vi "外观 2.vi"(0 "Data In":T5 caption="数据输入", 2 "Display State In":T3 caption="显示状态输入", 3 "Container State":T4 caption="容器状态") -> (6 "Data Out":T5 caption="数据输出", 7 "Display State Out":T3 caption="显示状态输出", 8 "Action":T2 caption="动作")   [LabVIEW 2016, in "运维调试菜单_古田户外.xctl"]
uses:
  <vilib>/_xctls/Container State.ctl
  <vilib>/_xctls/Action.ctl
  <vilib>/_xctls/XControlSupport.lvlib
panel:
  in  "单选按钮":T1(radio)
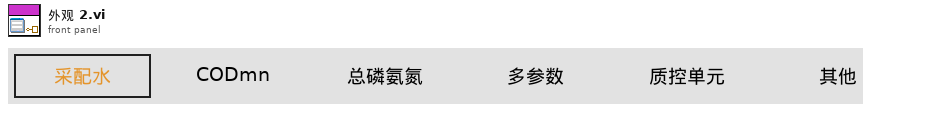
[diagram p1: front panel]
types:
  T1 = enum32{"采配水", "CODMn", "总磷氨氮", "pH", "质控单元", "其他"}
  T2 = typedef "XControlSupport.lvlib/Action.ctl" = cluster{"Data Changed?":bool, "State Changed?":bool, "Action Name":string}
  T3 = typedef "运维调试菜单_古田户外.xctl/状态 2.ctl" = cluster{"Numeric":dbl}
  T4 = typedef "XControlSupport.lvlib/Container State.ctl" = cluster{"Indicator?":bool, "Run Mode?":bool, " Refnum":refnum<vi>}
  T5 = typedef "运维调试菜单_古田户外.xctl/数据 2.ctl" = enum16{"采配水", "CODmn", "总磷氨氮", "多参数", "质控单元", "其他"}
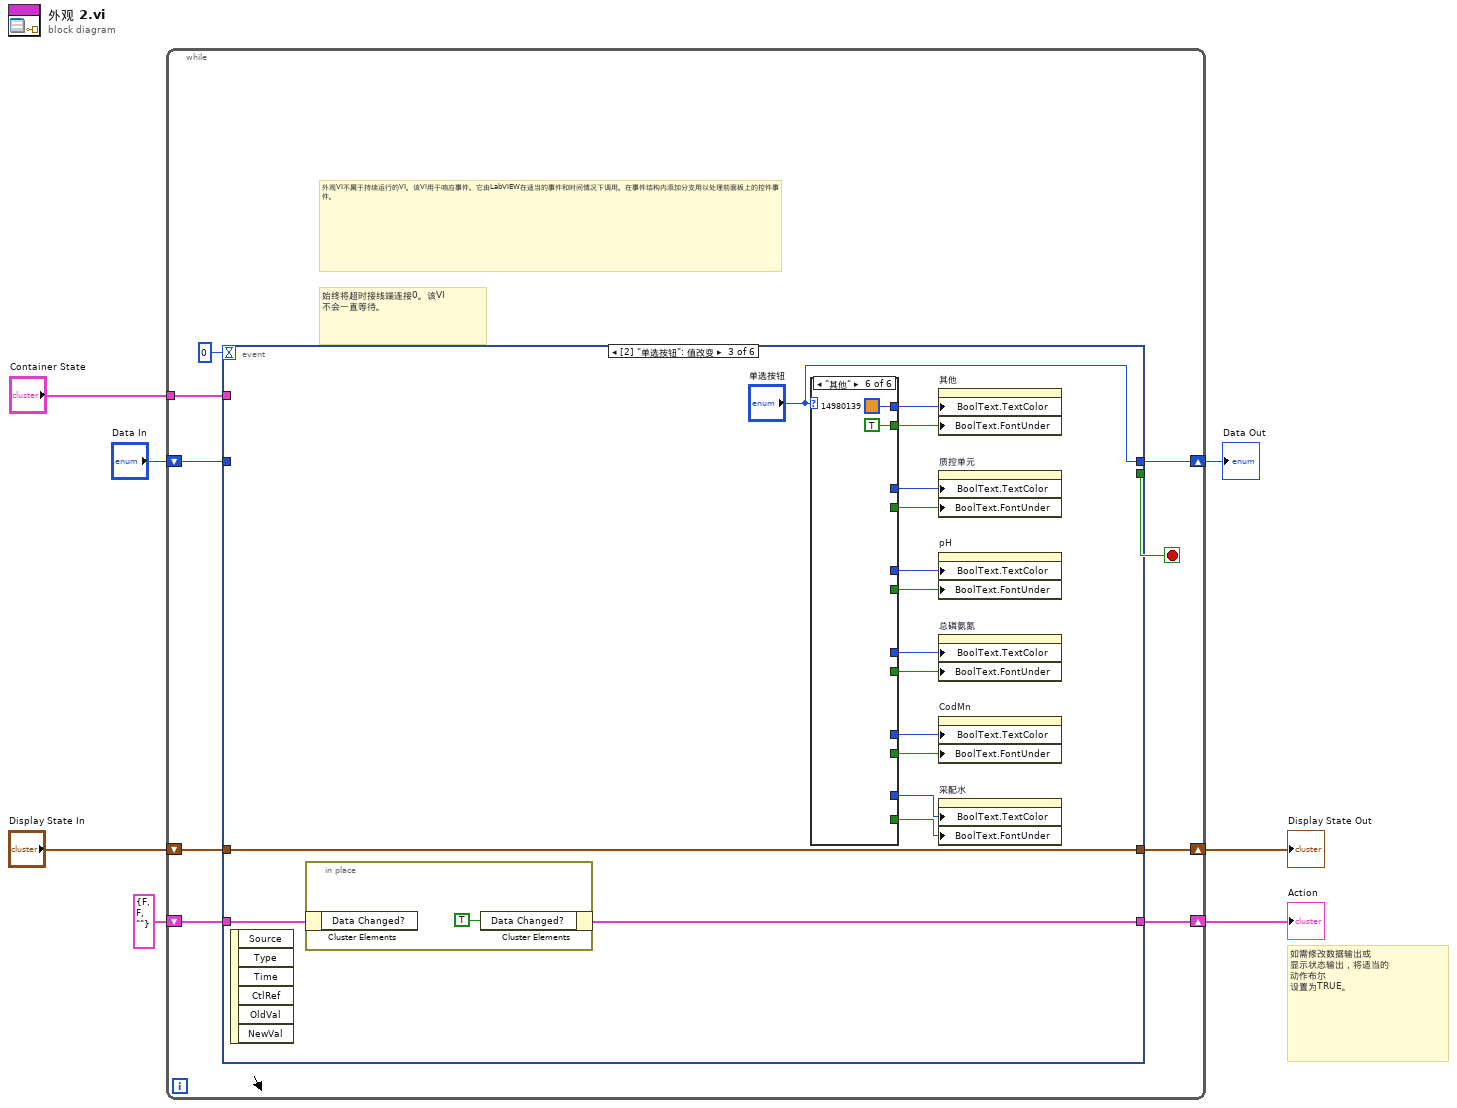
[diagram p0: block diagram]
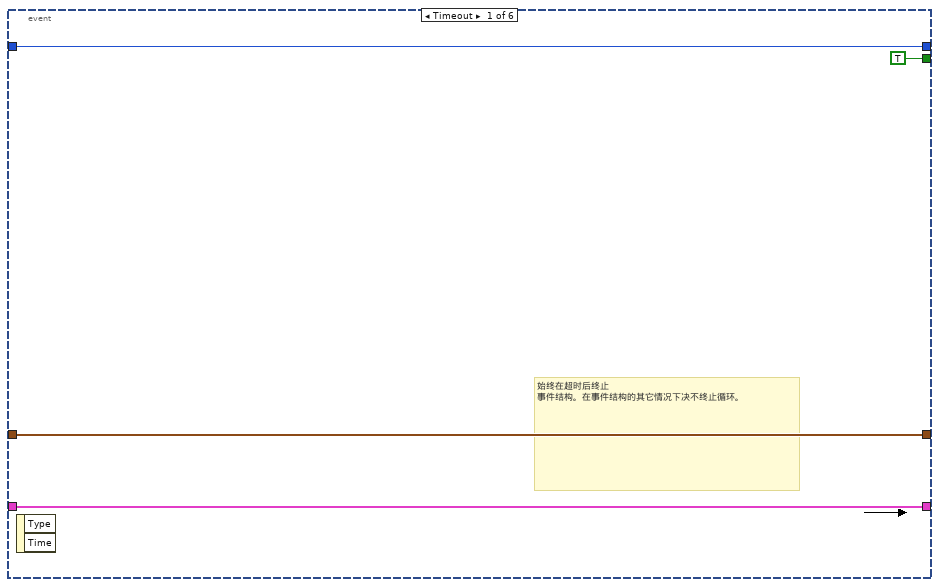
[diagram p2: hidden frame]
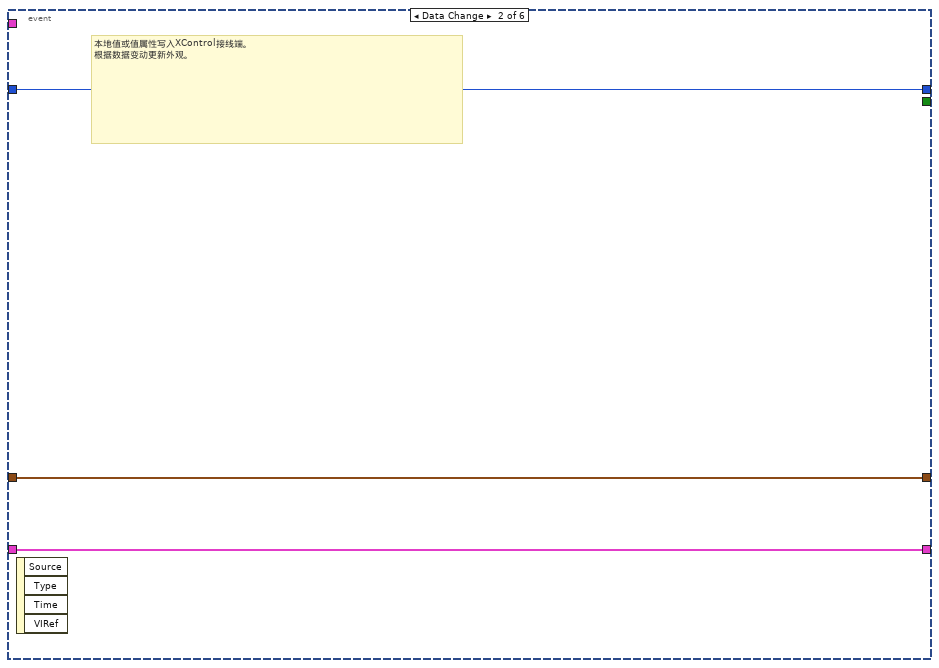
[diagram p3: hidden frame]
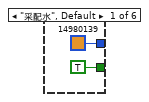
[diagram p4: hidden frame]
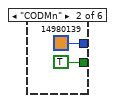
[diagram p5: hidden frame]
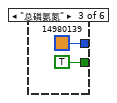
[diagram p6: hidden frame]
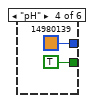
[diagram p7: hidden frame]
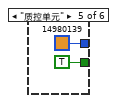
[diagram p8: hidden frame]
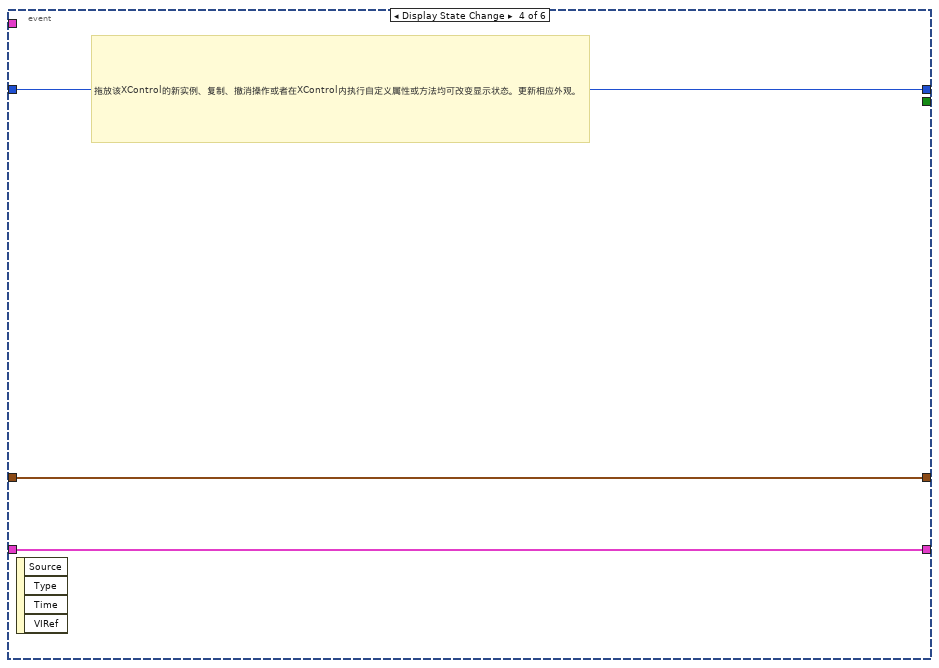
[diagram p9: hidden frame]
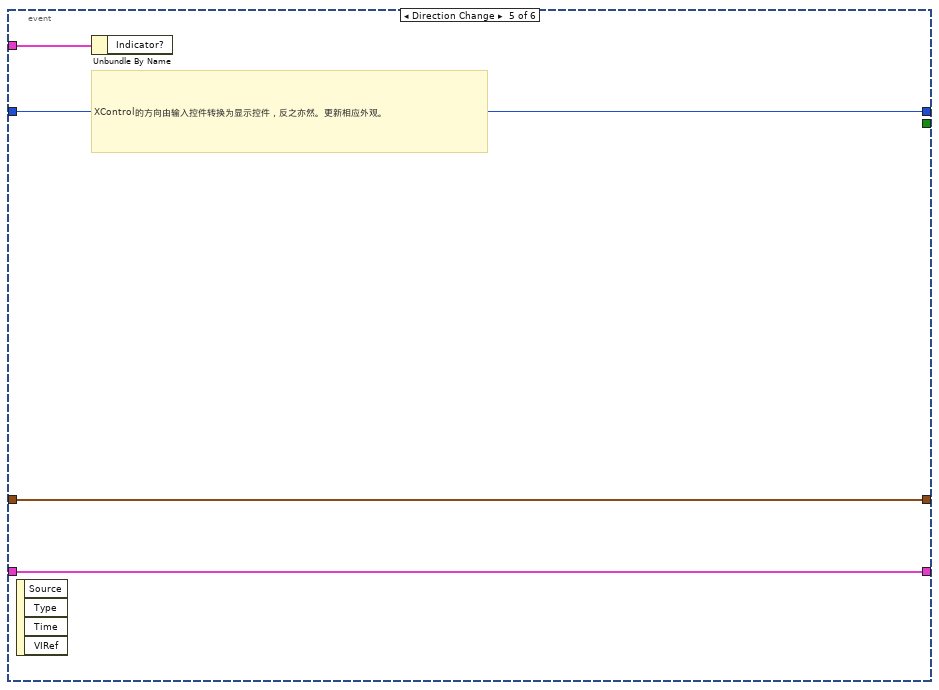
[diagram p10: hidden frame]
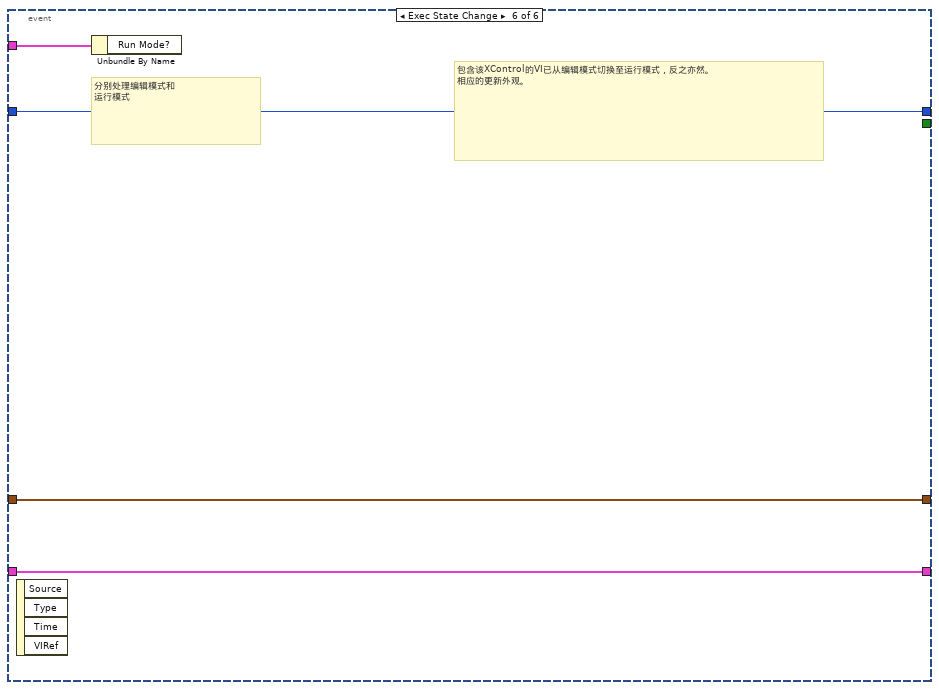
[diagram p11: hidden frame]
diagram:
  # "如需修改数据输出或\n显示状态输出，将适当的\n动作布尔\n设置为TRUE。"
  n1 = while {
    shift-right: [w15] -> w4
    shift-left: "Display State In" -> [w16]
    tunnel: "Container State" -> [w12]
    shift-right: [w10] -> w7
    shift-left: "Data In" -> [w11]
    shift-right: [w8] -> w2
    shift-left: T2 {"Data Changed?"=FALSE, "State Changed?"=FALSE, "Action Name"=""} ("Action") -> [w9]
    stop <- w14 stop-if-true
    # "外观VI不属于持续运行的VI。该VI用于响应事件。它由LabVIEW在适当的事件和时间情况下调用。在事件结构内添加分支用以处理前面板上的控件事件。"
    # "始终将超时接线端连接0。该VI\n不会一直等待。"
    n2 = event shown="[2] \"单选按钮\": 值改变" {
      selector: _ -> [_ _ _ _ _ _]
      dyn-events: _ -> [_ _ _ _ _ _]
      timeout: 0 -> [_ _ _ _ _ _]
      tunnel: w16 -> [w18 w22 w39 w55 w58 w62]
      tunnel: [w18 w22 w39 w55 w58 w62] -> w15
      tunnel: [TRUE _ _ _ _ _] -> w14
      tunnel: w12 -> [_ _ _ _ w59 w63]
      tunnel: w11 -> [w17 w23 _ w54 w57 w61]
      tunnel: [w17 w23 "单选按钮" w54 w57 w61] -> w10
      tunnel: [w19 w21 w37 w53 w56 w60] -> w8
      tunnel: w9 -> [w19 w21 w38 w53 w56 w60]
      event Timeout {
        # "始终在超时后终止\n事件结构。在事件结构的其它情况下决不终止循环。"
        n3 = event-data() -> ()  [unwired: 1 in, 2 out]
      }
      event Data Change {
        # "本地值或值属性写入XControl接线端。\n根据数据变动更新外观。"
        n4 = event-data() -> ()  [unwired: 1 in, 4 out]
      }
      event "单选按钮": Value Change {
        n5 = event-data() -> ()  [unwired: 1 in, 6 out]
        n6 = in-place {
          n7 = in-place-cluster #1(w38) -> ()  [unwired: 1 out]
          n8 = in-place-cluster #1("Data Changed?"=TRUE) -> (w37:T2)
        }
        n9 = case shown="\"其他\"" "单选按钮" {
          tunnel: [u32 14980139 _ _ _ _ _] -> w35
          tunnel: [TRUE ("布尔文本.字体:下划线") _ _ _ _ _] -> w34
          tunnel: [_ u32 14980139 _ _ _ _] -> w33
          tunnel: [_ TRUE ("布尔文本.字体:下划线") _ _ _ _] -> w32
          tunnel: [_ _ u32 14980139 _ _ _] -> w31
          tunnel: [_ _ TRUE ("布尔文本.字体:下划线") _ _ _] -> w30
          tunnel: [_ _ _ u32 14980139 _ _] -> w29
          tunnel: [_ _ _ TRUE ("布尔文本.字体:下划线") _ _] -> w28
          tunnel: [_ _ _ _ u32 14980139 _] -> w27
          tunnel: [_ _ _ _ TRUE ("布尔文本.字体:下划线") _] -> w26
          tunnel: [_ _ _ _ _ u32 14980139] -> w25
          tunnel: [_ _ _ _ _ TRUE ("布尔文本.字体:下划线")] -> w24
          frame "采配水", Default {
          }
          frame "CODMn" {
          }
          frame "总磷氨氮" {
          }
          frame "pH" {
          }
          frame "质控单元" {
          }
          frame "其他" {
          }
        }
        n10 = property on="其他" class="Bool (严格)"("BoolText.TextColor"=w25, "BoolText.FontUnder"=w24) -> ()  [unwired: 2 in, 2 out]
        n11 = property on="质控单元" class="Bool (严格)"("BoolText.TextColor"=w27, "BoolText.FontUnder"=w26) -> ()  [unwired: 2 in, 2 out]
        n12 = property on="pH" class="Bool (严格)"("BoolText.TextColor"=w29, "BoolText.FontUnder"=w28) -> ()  [unwired: 2 in, 2 out]
        n13 = property on="总磷氨氮" class="Bool (严格)"("BoolText.TextColor"=w31, "BoolText.FontUnder"=w30) -> ()  [unwired: 2 in, 2 out]
        n14 = property on="CodMn" class="Bool (严格)"("BoolText.TextColor"=w33, "BoolText.FontUnder"=w32) -> ()  [unwired: 2 in, 2 out]
        n15 = property on="采配水" class="Bool (严格)"("BoolText.TextColor"=w35, "BoolText.FontUnder"=w34) -> ()  [unwired: 2 in, 2 out]
      }
      event Display State Change {
        # "拖放该XControl的新实例、复制、撤消操作或者在XControl内执行自定义属性或方法均可改变显示状态。更新相应外观。"
        n16 = event-data() -> ()  [unwired: 1 in, 4 out]
      }
      event Direction Change {
        # "XControl的方向由输入控件转换为显示控件，反之亦然。更新相应外观。"
        n17 = event-data() -> ()  [unwired: 1 in, 4 out]
        n18 = Unbundle By Name(w59) -> ()  [unwired: 1 out]
      }
      event Exec State Change {
        # "包含该XControl的VI已从编辑模式切换至运行模式，反之亦然。\n相应的更新外观。"
        # "分别处理编辑模式和\n运行模式"
        n19 = event-data() -> ()  [unwired: 1 in, 4 out]
        n20 = Unbundle By Name(w63) -> ()  [unwired: 1 out]
      }
    }
  }
  "Display State Out" <- w4
  "Data Out" <- w7
  "Action" <- w2
